vi "Range Maximum Read.vi"(6 "Control Ref Queue":T1, 8 "error in (no error)":errorcluster, 11 "3D Plot.lvclass in":refnum<class "3D Plot.lvclass">) -> (0 "error out":errorcluster, 1 "Range Max":sgl, 3 "3D Plot.lvclass out":refnum<class "3D Plot.lvclass">)   [LabVIEW 2020, in "3D Plot.lvclass"]
uses:
  <vilib>/Math Plots/3D Math Plots/3D Plot/3D Plot/3D Plot.lvclass
  <vilib>/Math Plots/3D Math Plots/3D Plot/Action String/3DMathPlot Ctrl Act Queue.ctl
  <vilib>/Math Plots/3D Math Plots/3D Plot/Action String/3DMathPlot Ctrl Act Cluster.ctl
  <vilib>/Math Plots/3D Math Plots/3D Plot/Action String/3DMathPlot State Class.ctl
  <vilib>/Math Plots/3D Math Plots/3D Plot/3D Plot/3D Plot.lvclass/3D Plot.ctl
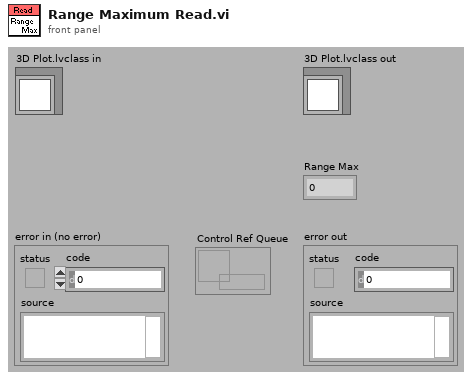
[diagram p1: front panel]
types:
  T1 = typedef "3DMathPlot Ctrl Act Queue.ctl" = refnum<queue>
  T2 = typedef "3D Plot.lvclass/Range Clusters.ctl" = cluster{"X Range":cluster{"Max X":sgl, "Min X":sgl}, "Y Range":cluster{"Max Y":sgl, "Min Y":sgl}, "Z Range":cluster{"Max Z":sgl, "Min Z":sgl}}
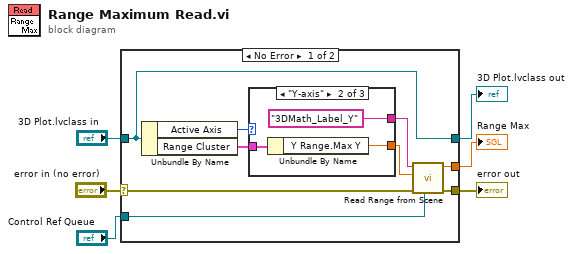
[diagram p0: block diagram]
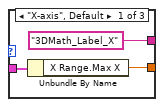
[diagram p2: hidden frame]
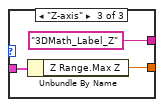
[diagram p3: hidden frame]
diagram:
  n1 = case shown="No Error" "error in (no error)" {
    selector: "error in (no error)" -> [w12 w25]
    tunnel: [w10 _] -> w6
    tunnel: "3D Plot.lvclass in" -> [w13 w26]
    tunnel: [w9 w25] -> w3
    tunnel: [w13 w26] -> w2
    tunnel: "Control Ref Queue" -> [w7 _]
    frame No Error {
      n2 = Unbundle By Name(w13) -> ("Active Axis"=w14:enum16{"X-axis", "Y-axis", "Z-axis"}, "Range Cluster"=w15:T2)
      n3 = case shown="\"Y-axis\"" w14 {
        tunnel: w15 -> [w17 w21 w24]
        tunnel: [w18 w20 w23] -> w11
        tunnel: ["3DMath_Label_X" "3DMath_Label_Y" ("Label Object Name") "3DMath_Label_Z" ("Label Object Name")] -> w8
        frame "X-axis", Default {
          n4 = Unbundle By Name(w17) -> ("X Range.Max X"=w18:sgl)
        }
        frame "Y-axis" {
          n5 = Unbundle By Name(w21) -> ("Y Range.Max Y"=w20:sgl)
        }
        frame "Z-axis" {
          n6 = Unbundle By Name(w24) -> ("Z Range.Max Z"=w23:sgl)
        }
      }
      n7 = call <vilib>:"Read Range from Scene.vi"("Control Ref Queue"=w7, "error in (no error)"=w12, "Default Range Value"=w11, "Label Object Name"=w8) -> ("error out"=w9:errorcluster, "Max"=w10:sgl)  [unwired: 5 in, 1 out]
    }
    frame Error {
    }
  }
  "error out" <- w3
  "Range Max" <- w6
  "3D Plot.lvclass out" <- w2
